vi "Tell Controller to Check Fcn and Dev Selection.vi"(8 "error in (no error)":errorcluster, 10 "Function Name":string, 11 "Controller UI in":refnum<class "Controller UI.lvclass">) -> (0 "error out":errorcluster, 3 "Controller UI out":refnum<class "Controller UI.lvclass">)   [LabVIEW 2016, in "Controller UI.lvlib" / "Controller UI.lvclass"]
uses:
  <userlib>/Common Components/Controller UI/Controller UI.lvclass
  C:/Program Files (x86)/National Instruments/LabVIEW 2016/vi.lib/ActorFramework/Actor/Actor.lvclass
  <userlib>/Common Components/Controller UI/Controller UI.lvclass/Controller UI.ctl
  <vilib>/ActorFramework/Actor/Actor.lvclass/Actor.ctl
  <userlib>/Common Components/Hardware/DevInfo/DevInfo.lvclass
  <userlib>/Common Components/Controller Messages/Check Fcn and Dev Selection requested by UI Msg/Check Fcn and Dev Selection requested by UI Msg.lvclass/Check Fcn and Dev Selection requested by UI Msg.ctl
  <vilib>/ActorFramework/Message Enqueuer/Message Enqueuer.lvclass/Message Enqueuer.ctl
  <vilib>/ActorFramework/Message Enqueuer/Enqueue.vi
  <userlib>/Common Components/Controller Messages/Check Fcn and Dev Selection requested by UI Msg/Check Fcn and Dev Selection requested by UI Msg.lvclass
  C:/Program Files (x86)/National Instruments/LabVIEW 2016/vi.lib/ActorFramework/Message/Message.lvclass
  <vilib>/ActorFramework/Message Priority Queue/Priority Enqueue.vi
  <vilib>/ActorFramework/Actor/Actor.lvclass
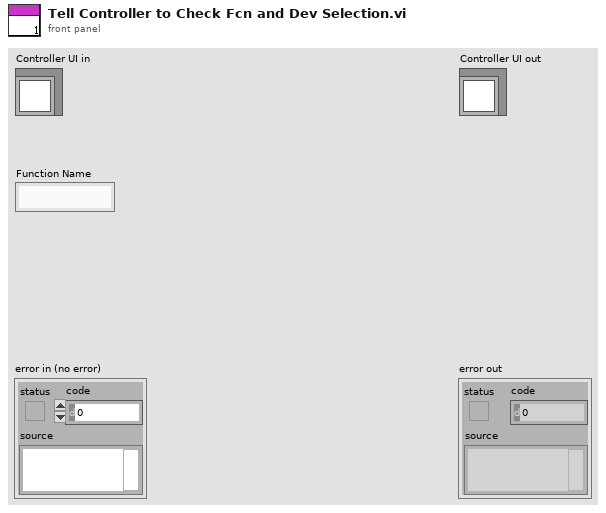
[diagram p1: front panel]
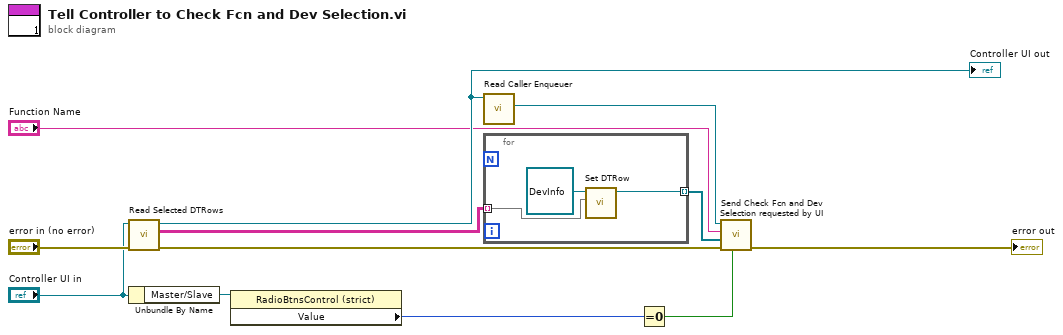
[diagram p0: block diagram]
diagram:
  n1 = call <userlib>:"Read Selected DTRows.vi"("error in (no error)"="error in (no error)", "Controller UI in"="Controller UI in") -> ("error out"=w6:errorcluster, "Selected DTRows"=w11:string[][], "Controller UI out"=w10:refnum<class "Controller UI.lvclass">)  [unwired: 7 in]
  "Controller UI out" <- w10
  n2 = Unbundle By Name("Controller UI in") -> ("Master/Slave"=w3:refnum<vi>)
  n3 = property class="RadioBtnsControl (strict)"(reference=w3) -> ("Value"=w2:enum32{"Master", "Slave"})  [unwired: 1 in, 2 out]
  n4 = call <vilib>:"Read Caller Enqueuer.vi"("Actor"=w10) -> ("Caller Enqueuer"=w9:refnum<class "Message Enqueuer.lvclass">)  [unwired: 10 in]
  n5 = for {
    tunnel: w11 -> [w14] mode=indexing
    tunnel: [w13] -> w8 mode=indexing
    n6 = call <userlib>:"Set DTRow.vi"("Dev Row Elements"=w14, "DevInfo in"=refnum<class "DevInfo.lvclass"> refnum) -> ("DevInfo out"=w13:refnum<class "DevInfo.lvclass">)  [unwired: 8 in, 1 out]
  }
  n7 = Equal To 0?(x=w2) -> (x = 0?=w1:bool)
  n8 = call <userlib>:"Send Check Fcn and Dev Selection requested by UI.vi"("Master?"=w1, "error in (no error)"=w6, "DevInfos"=w8, "Function Name"="Function Name", "Message Enqueuer"=w9) -> ("error out"=→"error out":errorcluster)  [unwired: 5 in, 1 out]
